vi "Logger_Time_Reset.vi"(11 "TDMS DevRef":T1) -> ()   [LabVIEW 2017]
uses:
  <userlib>/836-Library/System/TDMS_V2/Support/TDMS_DevRef.ctl
  <userlib>/836-Library/System/TDMS_V2/Support/Logging_Settings.ctl
  <userlib>/836-Library/System/TDMS_V2/Support/Group_FIFO_Config.ctl
  <userlib>/836-Library/System/TDMS_V2/Support/Channel_FIFO_Config.ctl
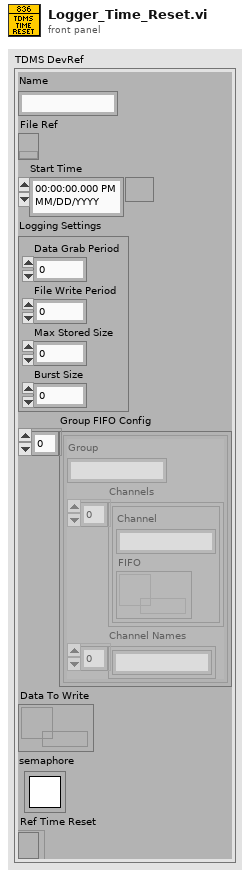
[diagram p1: front panel]
types:
  T1 = typedef "TDMS_DevRef.ctl" = cluster{"Name":string, "File Ref":refnum<k34>, "Start Time":timestamp, "Logging Settings":T2, "Group FIFO Config":T3[], "Data To Write":refnum<data-value>, "semaphore":T5, "Ref Time Reset":refnum<k4>}
  T2 = typedef "Logging_Settings.ctl" = cluster{"Data Grab Period":dbl, "File Write Period":dbl, "Max Stored Size":dbl, "Burst Size":dbl}
  T3 = typedef "Group_FIFO_Config.ctl" = cluster{"Group":string, "Channels":T4[], "Channel Names":string[]}
  T4 = typedef "Channel_FIFO_Config.ctl" = cluster{"Channel":string, "FIFO":refnum<k33>}
  T5 = typedef "Semaphore RefNum" = refnum<k1>
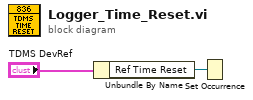
[diagram p0: block diagram]
diagram:
  n1 = Unbundle By Name("TDMS DevRef") -> ("Ref Time Reset"=w1:refnum<k4>)
  n2 = Set Occurrence(w1) -> ()
